vi "poc.ip.test.vi"() -> ()   [LabVIEW 2025]
uses:
  <vilib>/Platform/TimedLoop/XDataNode/XDataNode.xnode
  <vilib>/Platform/TimedLoop/XDataNode/nitl_modes.ctl
  <vilib>/Platform/TimedLoop/XDataNode/XDNodeRunTimeDep.lvlib
  <vilib>/Platform/TimedLoop/XDataNode/wakeup.ctl
  <vilib>/Platform/TimedLoop/XDataNode/timing_clust.ctl
  <vilib>/rvi/DataTransferAndStorage/Container/XNode/niFpgaContainer.xnode
  <vilib>/rvi/interface/RandomDataEmulation/nirviRandomDataFpgaMultiElementTemplate.vi
  <vilib>/rvi/LocalResourceManager/LocalResourceManager.xnode
  axi_2_eth_raw.ctl
  <vilib>/rvi/FIFO/Fifo_Resource/niFpgaFifoEmulationRefIn.vi
  <vilib>/rvi/DataTransferAndStorage/Container/Common/niFpgaContainerGetUniqueNameForEmu.vi
  <vilib>/rvi/DataTransferAndStorage/Container/Common/niFpgaContainerSetEmuInfo.vi
  <vilib>/rvi/eio/common/nirviEmuReportErrorAndStop.vi
  <vilib>/rvi/Memory/Memory_Emulation/niFpgaMemoryEmulationRefIn.vi
  submodules/Market.Data.Common/fpga/fpganow.common.fpga.lvlib
  submodules/Market.Data.Bats.Parser/fpga/poc.ip.axi.write.states.ctl
  <vilib>/rvi/FIFO/Fifo_Resource/nirvififoEmulationRead.vi
panel:
  in  "ip.Reset":bool
  out "i":u16
  out "Data":T1
  out "Numeric":i32
  in  "Reset":bool
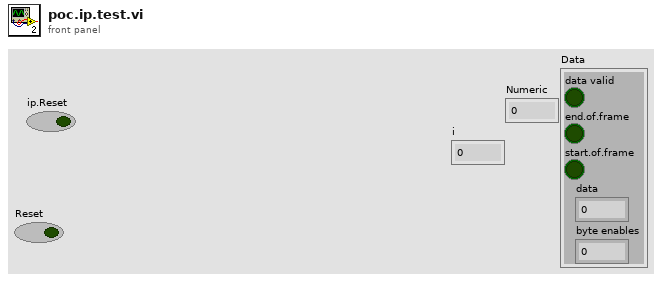
[diagram p1: front panel]
types:
  T1 = cluster{"data valid":bool, "end.of.frame":bool, "start.of.frame":bool, "data":u64, "byte enables":u8}
  T2 = typedef "XDNodeRunTimeDep.lvlib/timing_clust.ctl" = cluster{"Expected End [f-1]":u64, "Actual End [f-1]":u64, "Finished Late? [f-1]":bool, "Expected End [i-1]":u64, "Actual End [i-1]":u64, "Finished Late? [i-1]":bool, "Expected Start [i]":u64, "Actual Start [i]":u64, "Expected Start [f]":u64, "Actual Start [f]":u64, "Source Name":string, "Structure Name":string, "Period":i64, "Deadline":i64, "Offset":i64, "Start":i64, "Priority":i32, "Timeout":i32, "Mode":T3, "Wakeup Reason":T4, "Error":errorcluster, "Source Type":string, "Secondary Source Type":string, "Global End Time":u64, "Global Start Time":u64, "Frame Duration":u64, "Iteration Duration":u64, "Assigned CPU":i32, "I/O Scan Engine Mode":u32}
  T3 = typedef "XDNodeRunTimeDep.lvlib/nitl_modes.ctl" = enum32{"No Change", "Process missed periods, maintain original phase", "Discard missed periods, maintain original phase", "Process missed periods, ignore original phase", "Discard missed periods, ignore original phase"}
  T4 = typedef "XDNodeRunTimeDep.lvlib/wakeup.ctl" = enum32{"Normal", "Aborted", "Asynchronous wakeup", "Timing source error", "Timed loop error", "Timeout"}
  T5 = typedef "axi_2_eth_raw.ctl" = cluster{"data valid":bool, "end.of.frame":bool, "start.of.frame":bool, "data":u64, "byte enables":u8}
  T6 = cluster{"type":enum8{"Time", "AddOrder", "OrderExecuted", "OrderExecutedAtPrice", "ReduceSize", "ModifyOrder", "DeleteOrder", "Get.Everything", "Get.All.Orders", "Get.Top"}, "side":u8, "orderId ":u64, "quantity":u32, "symbol":u64, "price":u64, "executed.qty":u32, "canceled.qty":u32, "remaining.qty":u32, "seconds":u64, "nanoseconds":u64, "Add":bool, "Edit":bool, "Remove":bool, "seq no":u32, "recv.time":u64, "parse.time":u64}
  T7 = enum8{"Time", "AddOrder", "OrderExecuted", "OrderExecutedAtPrice", "ReduceSize", "ModifyOrder", "DeleteOrder", "Get.Everything", "Get.All.Orders", "Get.Top"}
  T8 = typedef "poc.ip.axi.write.states.ctl" = enum16{"Wait", "Collect"}
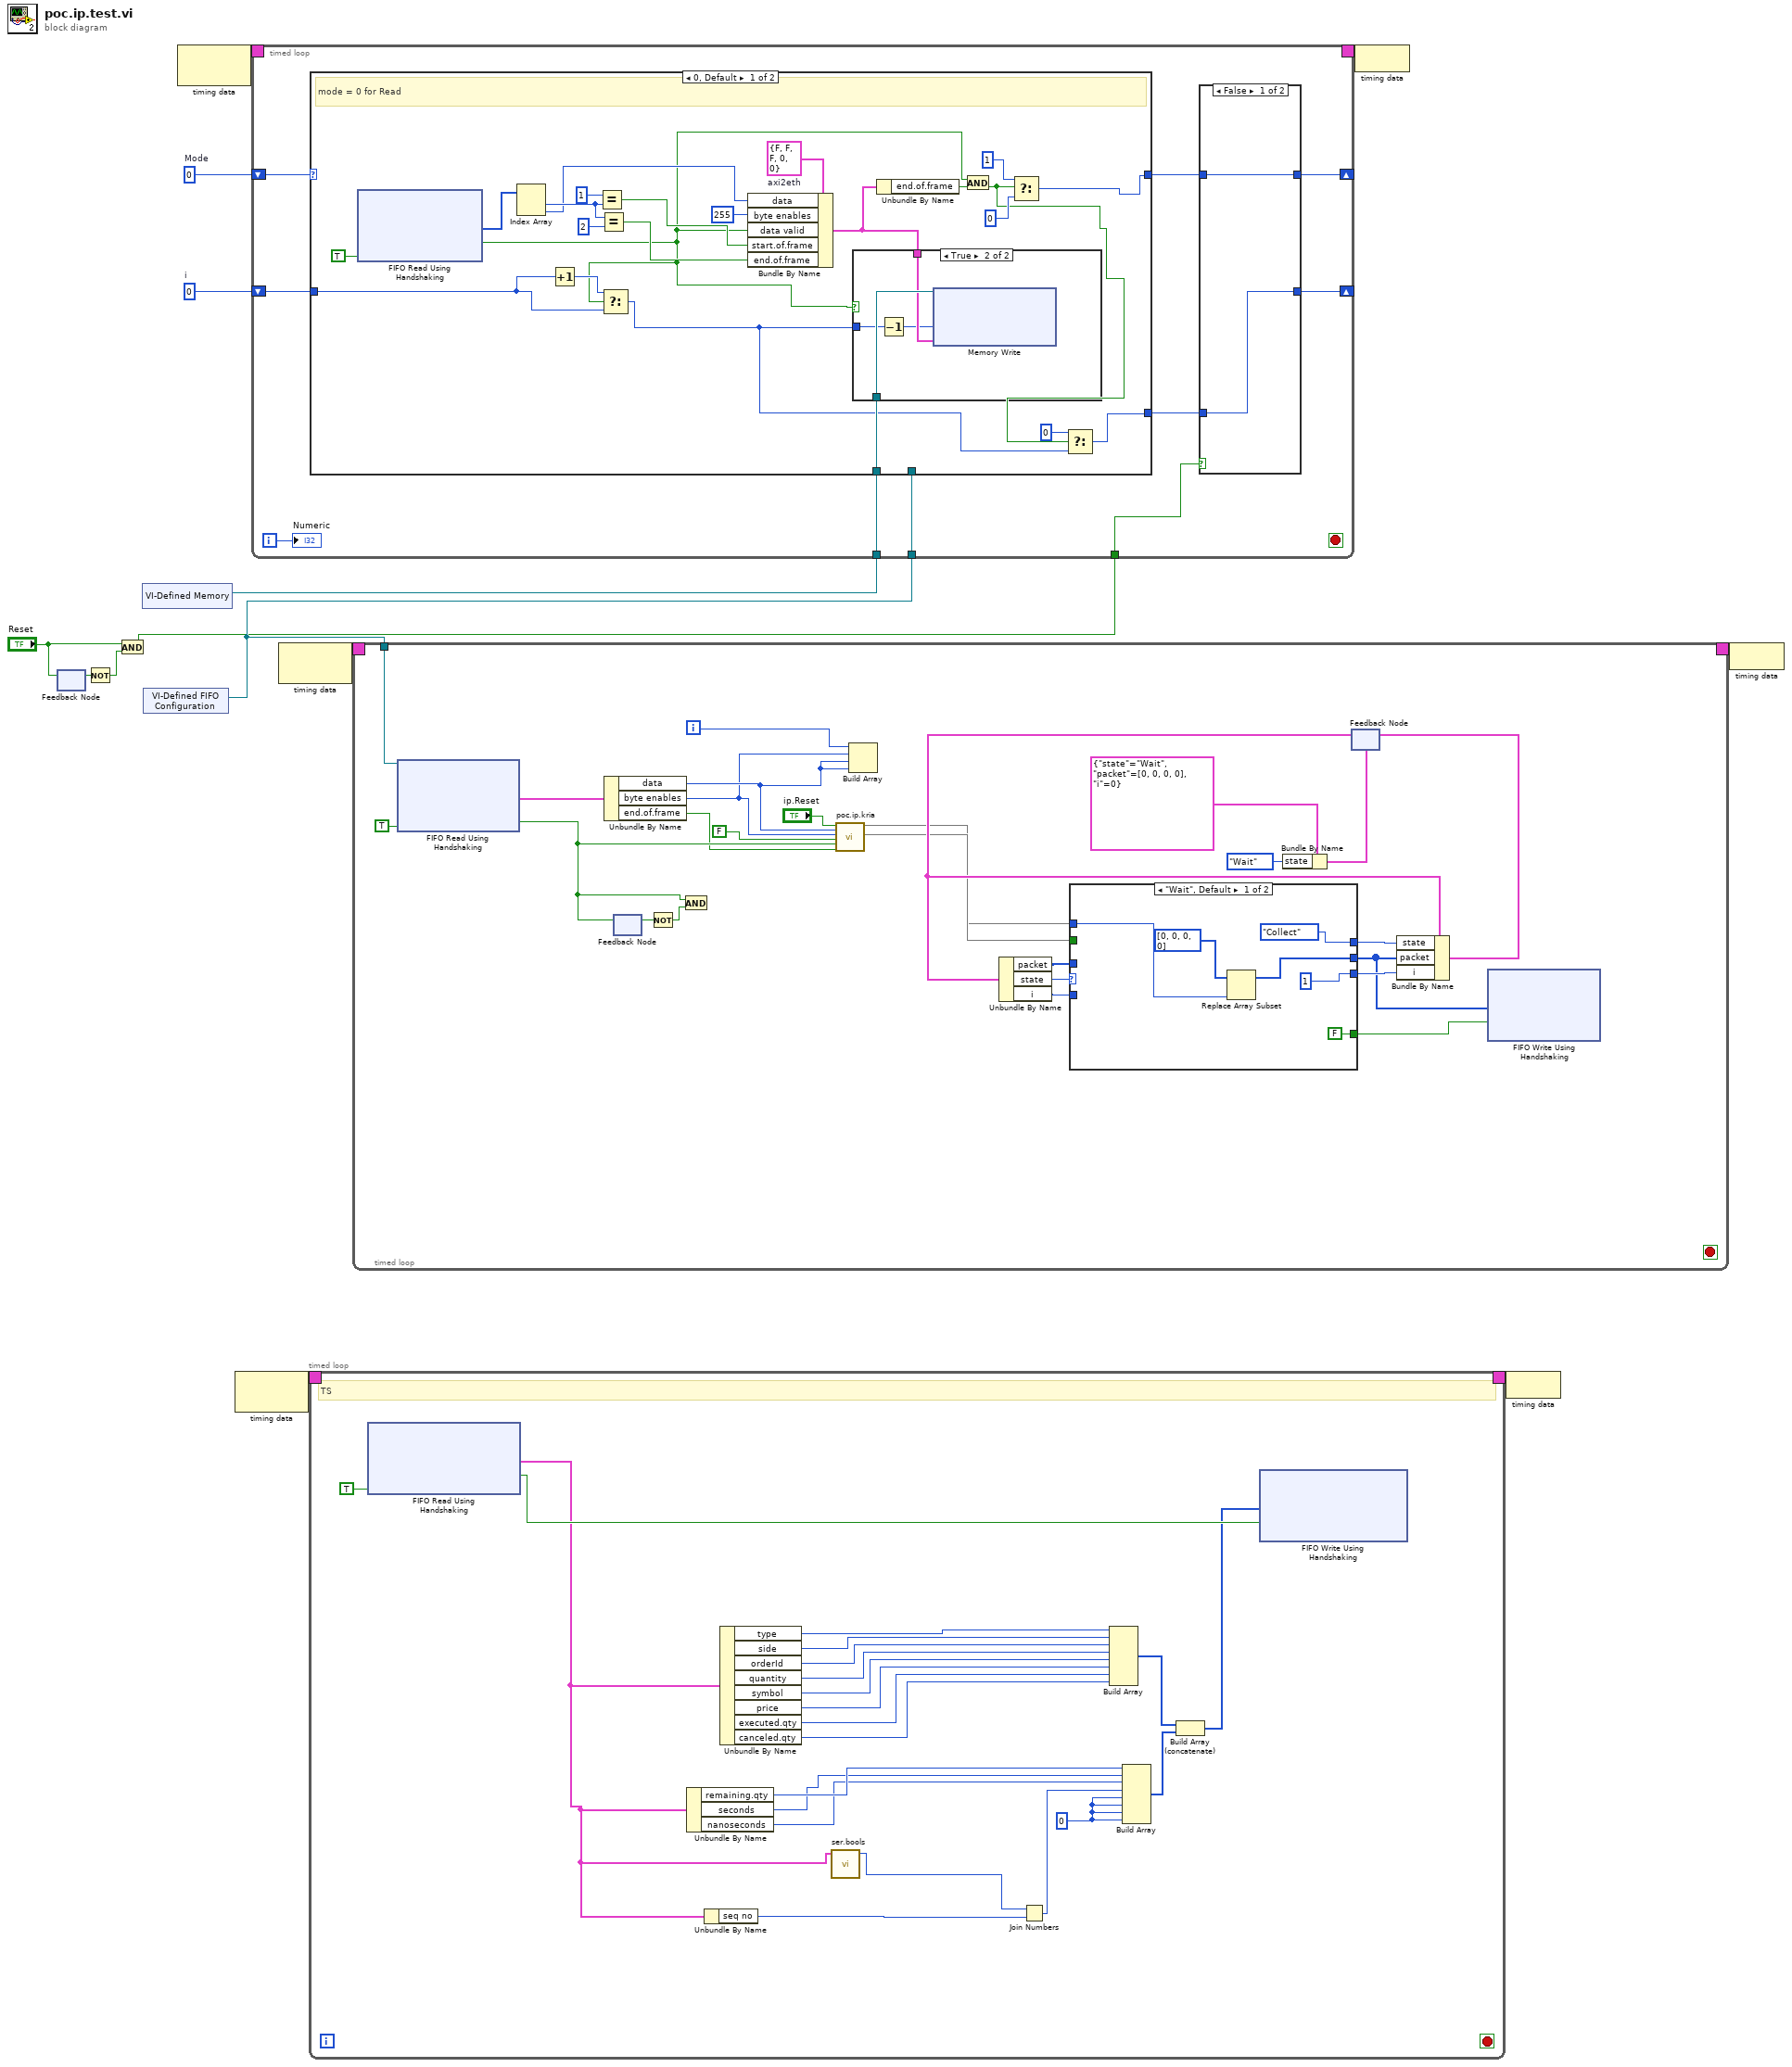
[diagram p0: block diagram]
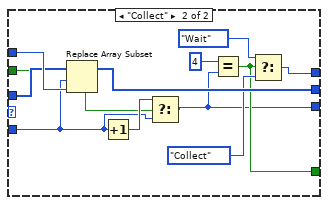
[diagram p2: hidden frame]
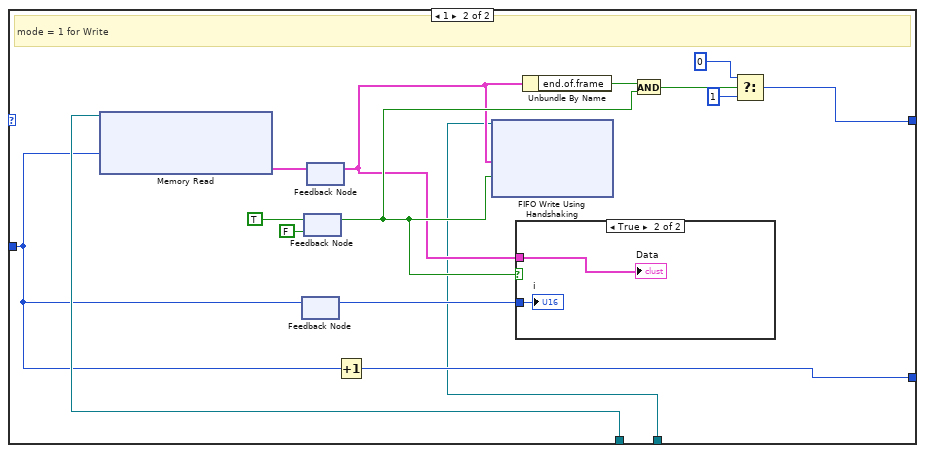
[diagram p4: hidden frame]
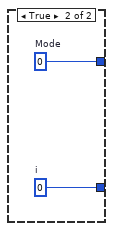
[diagram p6: hidden frame]
diagram:
  w4 = u16 0  # i
  w5 = u8 0  # Mode
  n1 = feedback-in #1("Reset") -> ()
  n2 = feedback #1() -> (w9:bool)  [unwired: 1 in]
  n3 = Not(x=w9) -> (.not. x?=w8:bool)
  n4 = And(x="Reset", y=w8) -> (x .and. y?=w6:bool)
  n5 = xnode "VI-Defined Memory"() -> ("Memory Out"=w3:refnum<k21>)
  n6 = xnode "VI-Defined FIFO Configuration"() -> ("FIFO Out"=w10:refnum<k21>)
  n7 = node-c288() -> (w14:T2)  [unwired: 1 in]
  n8 = node-c288() -> (w2:T2)  [unwired: 1 in]
  n9 = timed-loop {
    timing: w14 -> [_]
    timing-out: [_] -> w13
    tunnel: w10 -> [w16]
    tunnel: w6 -> [w19]
    shift-right: [w24] -> _
    shift-left: w5 -> [w23]
    shift-right: [w22] -> _
    shift-left: w4 -> [w21]
    tunnel: w3 -> [w20]
    i -> [w15]
    stop <- _ stop-if-true
    n10 = case shown="0, Default" w23 {
      tunnel: w21 -> [w36 w54]
      tunnel: w20 -> [w35 w66]
      tunnel: [w28 w60] -> w18
      tunnel: [w30 w63] -> w17
      tunnel: w16 -> [_ w52]
      frame 0, Default {
        w47 = T5 {"data valid"=FALSE, "end.of.frame"=FALSE, "start.of.frame"=FALSE, "data"=0, "byte enables"=0}  # axi2eth
        # "mode = 0 for Read"
        n11 = xnode "FIFO Read Using Handshaking"("Ready for Output"=TRUE) -> ("Element"=w46:u64[], "Output Valid"=w29:bool)  [unwired: 1 in, 1 out]
        n12 = Index Array(array=w46) -> (element #1=w45:u64, element #2=w39:u64)  [unwired: 2 in]
        n13 = Increment(x=w36) -> (x+1=w37:u16)
        n14 = Equal?(x=u64 1, y=w45) -> (x = y?=w41:bool)
        n15 = Equal?(x=w45, y=u64 2) -> (x = y?=w42:bool)
        n16 = Select(t=w37, s=w29, f=w36) -> (s? t:f=w27:u16)
        n17 = Bundle By Name(cluster=w47, "data"=w39, "byte enables"=u8 255 ("number"), "data valid"=w29, "start.of.frame"=w41, "end.of.frame"=w42) -> (w34:T5)
        n18 = case shown="True" w29 {
          tunnel: w35 -> [_ w51]
          tunnel: w34 -> [_ w50]
          tunnel: w27 -> [_ w49]
          frame False {
          }
          frame True {
            n19 = Decrement(x=w49) -> (x-1=w48:u16)
            n20 = xnode "Memory Write"("Address"=w48, "Data"=w50, "Memory In"=w51) -> ()  [unwired: 1 out]
          }
        }
        n21 = Unbundle By Name(w34) -> ("end.of.frame"=w33:bool)
        n22 = And(x=w29, y=w33) -> (x .and. y?=w26:bool)
        n23 = Select(t=u8 1, s=w26, f=u8 0 ("t")) -> (s? t:f=w30:u8)
        n24 = Select(t=u16 0, s=w26, f=w27) -> (s? t:f=w28:u16)
      }
      frame 1 {
        # "mode = 1 for Write"
        n25 = xnode "Memory Read"("Address"=w54, "Memory In"=w66) -> ("Data"=w65:T1)  [unwired: 1 out]
        n26 = feedback-in #2(w54) -> ()
        n27 = feedback #2() -> (w53:u16)  [unwired: 1 in]
        n28 = feedback-in #3(TRUE ("Input Valid")) -> ()
        n29 = feedback #3(FALSE ("Input Valid")) -> (w56:bool)
        n30 = feedback-in #4(w65) -> ()
        n31 = feedback #4() -> (w55:T1)  [unwired: 1 in]
        n32 = Increment(x=w54) -> (x+1=w60:u16)
        n33 = xnode "FIFO Write Using Handshaking"("Element"=w55, "Input Valid"=w56, "FIFO In"=w52) -> ()  [unwired: 2 out]
        n34 = case shown="True" w56 {
          tunnel: w55 -> [_ w68]
          tunnel: w53 -> [_ w67]
          frame False {
          }
          frame True {
            "Data" <- w68
            "i" <- w67
          }
        }
        n35 = Unbundle By Name(w55) -> ("end.of.frame"=w64:bool)
        n36 = And(x=w64, y=w56) -> (x .and. y?=w57:bool)
        n37 = Select(t=u8 0 ("f"), s=w57, f=u8 1) -> (s? t:f=w63:u8)
      }
    }
    n38 = case shown="False" w19 {
      tunnel: [w69 w72] -> w24
      tunnel: [w70 w71] -> w22
      tunnel: w18 -> [w70 _]
      tunnel: w17 -> [w69 _]
      frame False {
      }
      frame True {
        w71 = u16 0  # i
        w72 = u8 0  # Mode
      }
    }
    "Numeric" <- w15
  }
  n39 = node-c288() -> (w12:T2)  [unwired: 1 in]
  n40 = timed-loop {
    timing: w2 -> [_]
    timing-out: [_] -> w1
    stop <- _ stop-if-true
    w82 = u64 0 ("element")
    # "TS"
    n41 = xnode "FIFO Read Using Handshaking"("Ready for Output"=TRUE) -> ("Element"=w75:T6, "Output Valid"=w94:bool)  [unwired: 1 in, 1 out]
    n42 = Unbundle By Name(w75) -> ("remaining.qty"=w83:u32, "seconds"=w80:u64, "nanoseconds"=w81:u64)
    n43 = Unbundle By Name(w75) -> ("seq no"=w78:u32)
    n44 = Unbundle By Name(w75) -> ("type"=w93:T7, "side"=w92:u8, "orderId"=w91:u64, "quantity"=w90:u32, "symbol"=w89:u64, "price"=w88:u64, "executed.qty"=w87:u32, "canceled.qty"=w86:u32)
    n45 = call "ser.bools.vi"("orderbook.command"=w75) -> ("Numeric"=w76:u32)  [unwired: 10 in]
    n46 = Join Numbers(hi=w76, lo=w78) -> ((hi.lo)=w79:u64)
    n47 = Build Array(w93, w92, w91, w90, w89, w88, w87, w86) -> (w85:u64[])
    n48 = Build Array(w83, w80, w81, w79, w82, w82, w82, w82) -> (w84:u64[])
    n49 = Build Array (concatenate)(w85, w84) -> (w77:u64[])
    n50 = xnode "FIFO Write Using Handshaking"("Element"=w77, "Input Valid"=w94) -> ()  [unwired: 1 in, 2 out]
  }
  n51 = timed-loop {
    timing: w12 -> [_]
    timing-out: [_] -> w11
    tunnel: w10 -> [w123]
    i -> [w120]
    stop <- _ stop-if-true
    n52 = xnode "FIFO Read Using Handshaking"("Ready for Output"=TRUE, "FIFO In"=w123) -> ("Element"=w121:T1, "Output Valid"=w119:bool)  [unwired: 1 out]
    n53 = Unbundle By Name(w121) -> ("data"=w115:u64, "byte enables"=w114:u8, "end.of.frame"=w112:bool)
    n54 = feedback #5() -> (w118:bool)  [unwired: 1 in]
    n55 = feedback-in #5(w119) -> ()
    n56 = Not(x=w118) -> (.not. x?=w117:bool)
    n57 = And(x=w119, y=w117) -> ()  [unwired: 1 out]
    n58 = call "poc.ip.kria.vi"("ip.reset"="ip.Reset", "TDATA"=w115, "TKEEP"=w114, "TUSER"=FALSE, "TVALID"=w119, "TLAST"=w112) -> (14:w102, 16:w103)  [unwired: 12 in]
    n59 = Build Array(w120, w114, w115, w115) -> ()  [unwired: 1 out]
    n60 = Bundle By Name(cluster=cluster{"state":T8, "packet":u64[], "i":u16} {"state"=enum."Wait", "packet"=[0, 0, 0, 0], "i"=0}, "state"=poc.ip.axi.write.states."Wait" ("Enum")) -> (w107:cluster{"state":T8, "packet":u64[], "i":u16})
    n61 = feedback #6(w107) -> (w106:cluster{"state":T8, "packet":u64[], "i":u16})
    n62 = Unbundle By Name(w106) -> ("packet"=w99:u64[], "state"=w110:T8, "i"=w100:u16)
    n63 = case shown="\"Wait\", Default" w110 {
      tunnel: [FALSE w135] -> w109
      tunnel: [poc.ip.axi.write.states."Collect" ("state") w134] -> w104
      tunnel: w103 -> [_ w131]
      tunnel: w102 -> [w125 w141]
      tunnel: [u16 1 ("i") w130] -> w101
      tunnel: [w124 w139] -> w98
      tunnel: w100 -> [_ w132]
      tunnel: w99 -> [_ w140]
      frame "Wait", Default {
        n64 = Replace Array Subset(array=u64[] [0, 0, 0, 0] ("packet"), new element=w125) -> (w124:u64[])  [unwired: 1 in]
      }
      frame "Collect" {
        n65 = Replace Array Subset(array=w140, new element=w141, index=w132) -> (w139:u64[])
        n66 = Increment(x=w132) -> (x+1=w133:u16)
        n67 = Select(t=w133, s=w131, f=w132) -> (s? t:f=w130:u16)
        n68 = Equal?(x=u16 4, y=w130) -> (x = y?=w135:bool)
        n69 = Select(t=poc.ip.axi.write.states."Wait" ("Enum"), s=w135, f=poc.ip.axi.write.states."Collect" ("Enum")) -> (s? t:f=w134:T8)
      }
    }
    n70 = Bundle By Name(cluster=w106, "state"=w104, "packet"=w98, "i"=w101) -> (w105:cluster{"state":T8, "packet":u64[], "i":u16})
    n71 = feedback-in #6(w105) -> ()
    n72 = xnode "FIFO Write Using Handshaking"("Element"=w98, "Input Valid"=w109) -> ()  [unwired: 1 in, 2 out]
  }
  n73 = node-c288(w13) -> ()
  n74 = node-c288(w1) -> ()
  n75 = node-c288(w11) -> ()
